vi "Calculate Resistance Specs.vi"(8 "Tol %":dbl, 11 "Nom Value":dbl) -> (0 "Tol Range":dbl, 1 "Desviation":dbl, 2 "Lower Limit":dbl, 3 "Upper Limit":dbl)   [LabVIEW 2018]
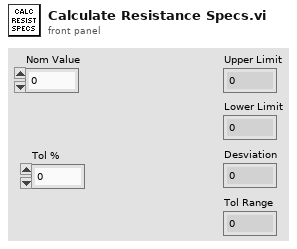
[diagram p1: front panel]
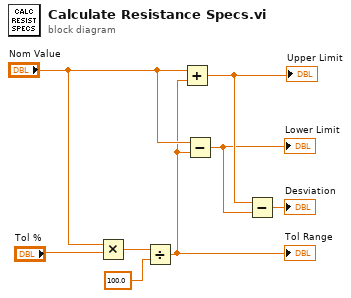
[diagram p0: block diagram]
diagram:
  n1 = Multiply(x="Nom Value", y="Tol %") -> (x*y=w7:dbl)
  n2 = Divide(x=w7, y=100.0) -> (x/y=w1:dbl)
  "Tol Range" <- w1
  n3 = Add(x="Nom Value", y=w1) -> (x+y=w4:dbl)
  "Upper Limit" <- w4
  n4 = Subtract(x="Nom Value", y=w1) -> (x-y=w3:dbl)
  "Lower Limit" <- w3
  n5 = Subtract(x=w4, y=w3) -> (x-y=→"Desviation":dbl)
